vi "Test Throw error on int type for bool.vi"(11 "Test Case In":refnum<class "Test Strict Find Items as LV Type.lvclass">) -> (0 "error out":errorcluster, 3 "Test Case Out":refnum<class "Test Strict Find Items as LV Type.lvclass">)   [LabVIEW 2024, in "Test Strict Find Items as LV Type.lvclass"]
uses:
  Test Strict Find Items as LV Type.lvclass
  Test Strict Find Items as LV Type.lvclass/Test Strict Find Items as LV Type.ctl
  7860c969-8ea9-4e34-a02d-68fc78db45ce.vi
  <vilib>/Astemes/LUnit/Test Case.lvclass
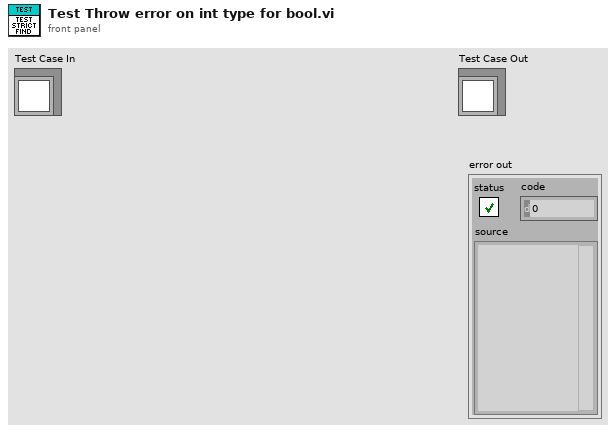
[diagram p1: front panel]
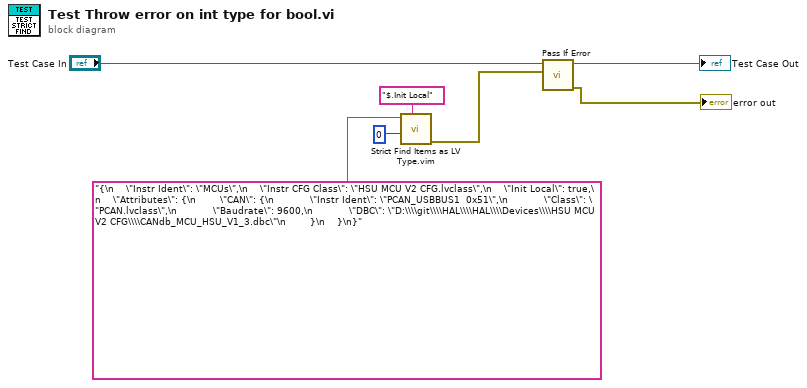
[diagram p0: block diagram]
diagram:
  n1 = call "Strict Find Items as LV Type.vim"("$Path or Item Name"="$.Init Local", "Data Type and Default Value"=u16 0, "<JSON>"="{\n    \"Instr Ident\": \"MCUs\",\n    \"Instr CFG Class\": \"HSU MCU V2 CFG.lvclass\",\n    \"Init Local\": true,\n    \"Attributes\": {\n        \"CAN\": {\n            \"Instr Ident\": \"PCAN_USBBUS1  0x51\",\n            \"Class\": \"PCAN.lvclass\",\n            \"Baudrate\": 9600,\n            \"DBC\": \"D:\\\\git\\\\HAL\\\\HAL\\\\Devices\\\\HSU MCU V2 CFG\\\\CANdb_MCU_HSU_V1_3.dbc\"\n        }\n    }\n}") -> ("error out"=w1:errorcluster)  [unwired: 6 in, 2 out]
  n2 = call <vilib>:"Pass If Error.vi"("Assert error"=w1, "LUnit Test Case In"="Test Case In") -> ("error out"=→"error out":errorcluster, "LUnit Test Case Out"=→"Test Case Out":refnum<class "Test Strict Find Items as LV Type.lvclass">)  [unwired: 8 in]
